vi "Write Emit Status Messages.vi"(8 "error in (no error)":errorcluster, 10 "Emit Status Messages":bool, 11 "Pub Sub Message Channel in":refnum<class "Pub Sub Message Channel.lvclass">) -> (0 "error out":errorcluster, 3 "Pub Sub Message Channel out":refnum<class "Pub Sub Message Channel.lvclass">)   [LabVIEW 2020, in "Actor Pub Sub Channels.lvlib" / "Pub Sub Message Channel.lvclass"]
uses:
  Pub Sub Message Channel.lvclass
  Pub Sub Message Channel.lvclass/Pub Sub Message Channel.ctl
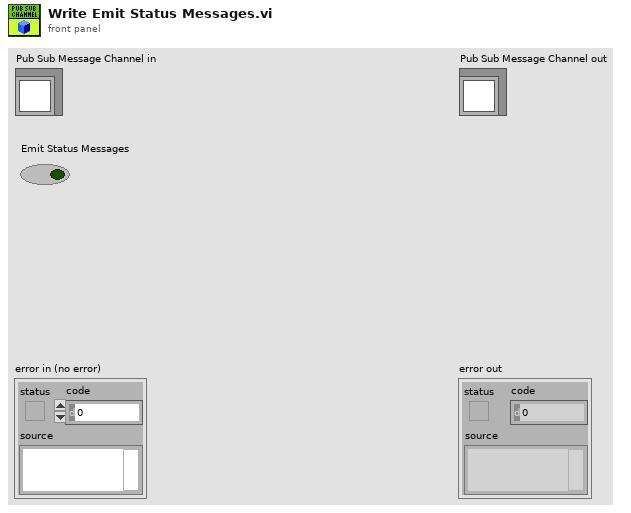
[diagram p1: front panel]
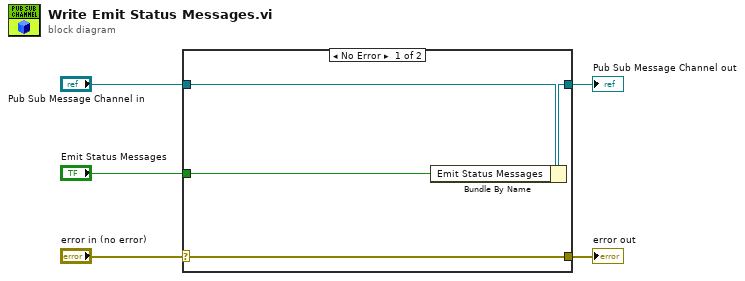
[diagram p0: block diagram]
diagram:
  n1 = case shown="No Error" "error in (no error)" {
    selector: "error in (no error)" -> [w9 w10]
    tunnel: [w9 w10] -> w4
    tunnel: [w7 w11] -> w2
    tunnel: "Pub Sub Message Channel in" -> [w8 w11]
    tunnel: "Emit Status Messages" -> [w6 _]
    frame No Error {
      n2 = Bundle By Name(cluster=w8, "Emit Status Messages"=w6) -> (w7:refnum<class "Pub Sub Message Channel.lvclass">)
    }
    frame Error {
    }
  }
  "error out" <- w4
  "Pub Sub Message Channel out" <- w2
